vi "Field Position.vi"() -> (0 "Field Angle":dbl, 1 "Field Y":dbl, 2 "Field X":dbl, 3 "Data Source":T1)   [LabVIEW 2013]
uses:
  Vision Tracking/Field Position Source.ctl
  Robot Global Data.vi
  <vilib>/Rock Robotics/WPI/Gyro/WPI_GyroRefNum Registry Get.vi
  <vilib>/Rock Robotics/WPI/Gyro/WPI_GyroGetAngle.vi
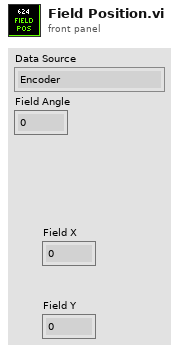
[diagram p1: front panel]
types:
  T1 = typedef "Field Position Source.ctl" = enum16{"Encoder", "Single Cam", "Dual Cam"}
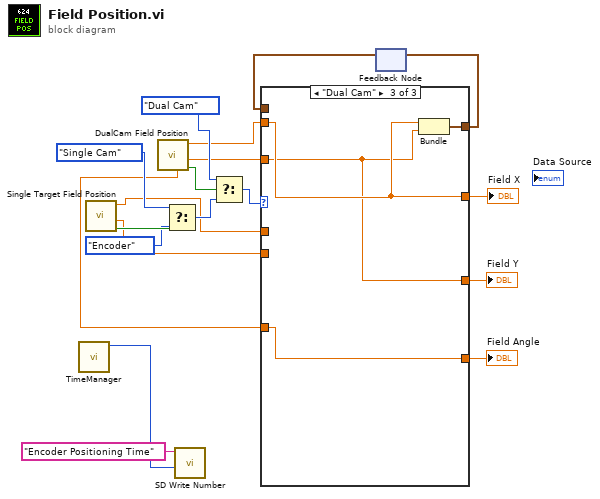
[diagram p0: block diagram]
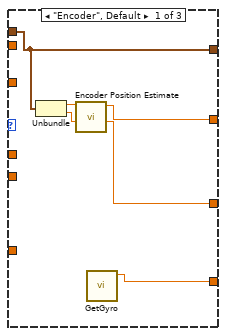
[diagram p2: hidden frame]
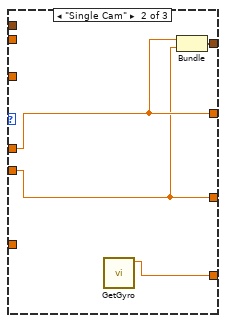
[diagram p3: hidden frame]
diagram:
  n1 = call "TimeManager.vi"() -> ("Time Since Reset"=w19:u32)  [unwired: 10 in, 1 out]
  n2 = call "Single Target Field Position.vi"() -> ("Goal Found?"=w14:bool, "Y"=w9:dbl, "X"=w10:dbl)  [unwired: 9 in]
  n3 = call "DualCam Field Position.vi"() -> ("Goal Found?"=w17:bool, "Y"=w5:dbl, "X"=w6:dbl, "Gyro Angle"=w1:dbl)  [unwired: 8 in]
  n4 = Select(t=Field_Position_Source."Single Cam" ("Data Source"), s=w14, f=Field_Position_Source."Encoder" ("Data Source")) -> (s? t:f=w15:T1)
  n5 = call <vilib>:"SD Write Number.vi"("Numeric"=w19, "Name"="Encoder Positioning Time") -> ()  [unwired: 8 in, 2 out]
  n6 = Select(t=Field_Position_Source."Dual Cam" ("Data Source"), s=w17, f=w15) -> (s? t:f=w11:T1)
  n7 = feedback #1() -> (w3:cluster{"X":dbl, "Y":dbl})  [unwired: 1 in]
  n8 = case shown="\"Dual Cam\"" w11 {
    tunnel: w10 -> [_ w29 _]
    tunnel: w9 -> [_ w28 _]
    tunnel: [w22 w29 w32] -> w8
    tunnel: [w21 w28 w31] -> w7
    tunnel: w6 -> [_ _ w32]
    tunnel: w5 -> [_ _ w31]
    tunnel: [w25 w27 w33] -> w4
    tunnel: w3 -> [w25 _ _]
    tunnel: [w20 w26 w30] -> w2
    tunnel: w1 -> [_ _ w30]
    frame "Encoder", Default {
      n9 = Unbundle(w25) -> ("X"=w24:dbl, "Y"=w23:dbl)
      n10 = call "Encoder Position Estimate.vi"("Last Vision Y"=w23, "Last Vision X"=w24) -> ("Y"=w21:dbl, "X"=w22:dbl)  [unwired: 8 in]
      n11 = call "GetGyro.vi"() -> ("Angle"=w20:dbl)  [unwired: 9 in, 2 out]
    }
    frame "Single Cam" {
      n12 = call "GetGyro.vi"() -> ("Angle"=w26:dbl)  [unwired: 9 in, 2 out]
      n13 = Bundle("X"=w29, "Y"=w28) -> (w27:cluster{"X":dbl, "Y":dbl})  [unwired: 1 in]
    }
    frame "Dual Cam" {
      n14 = Bundle("X"=w32, "Y"=w31) -> (w33:cluster{"X":dbl, "Y":dbl})  [unwired: 1 in]
    }
  }
  "Field X" <- w8
  "Field Y" <- w7
  "Field Angle" <- w2
  n15 = feedback-in #1(w4) -> ()
